vi "Create Process.vi"(8 "error in (no error)":errorcluster, 11 "Process Generator in":refnum<class "Process Generator.lvclass">) -> (0 "error out":errorcluster, 3 "Process Generator out":refnum<class "Process Generator.lvclass">)   [LabVIEW 2020, in "Process Generation.lvlib" / "Process Generator.lvclass"]
uses:
  Process Generator.lvclass
  Process Generator.lvclass/Process Generator.ctl
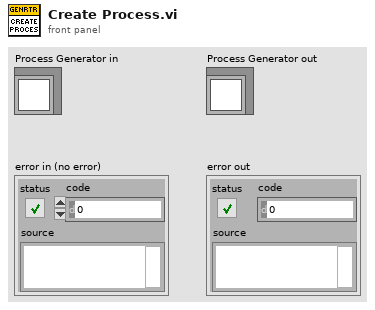
[diagram p1: front panel]
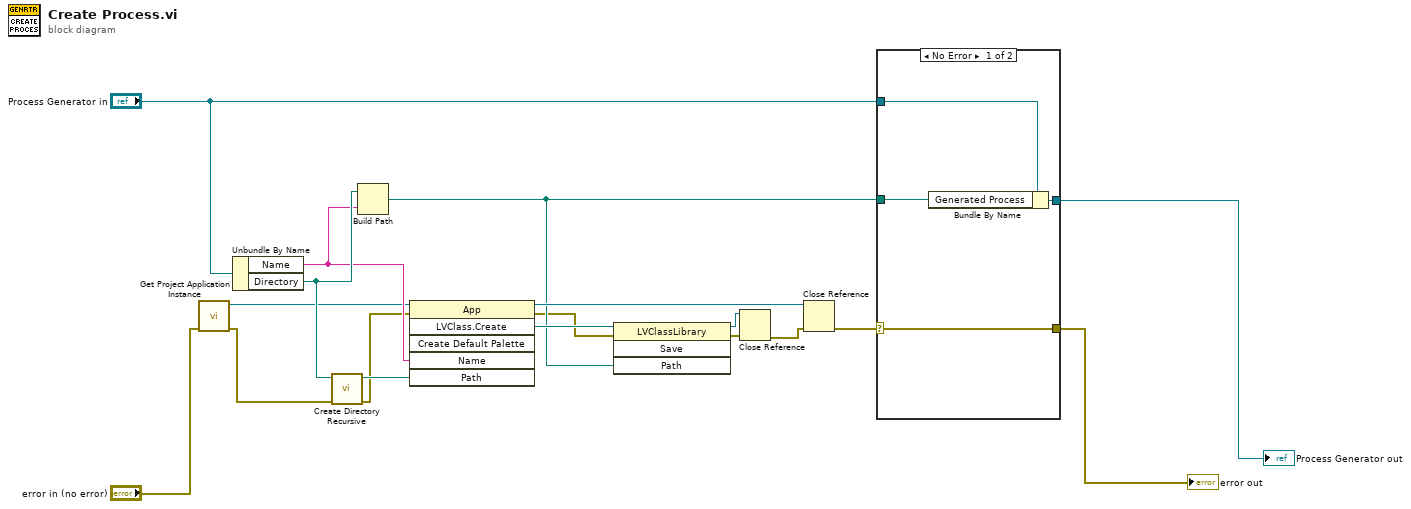
[diagram p0: block diagram]
diagram:
  n1 = call "Get Project Application Instance.vi"("error in (no error)"="error in (no error)") -> ("error out"=w10:errorcluster, "Application out"=w8:refnum<vi>)  [unwired: 9 in]
  n2 = Unbundle By Name("Process Generator in") -> ("Name"=w12:string, "Directory"=w13:path)
  n3 = call <vilib>:"Create Directory Recursive.vi"("error in (no error)"=w10, "directory"=w13) -> ("error out"=w7:errorcluster, "directory copy"=w18:path)  [unwired: 3 in, 1 out]
  n4 = Build Path(base path=w13, name or relative path=w12) -> (appended path=w5:path)
  n5 = invoke class="App" method="LVClass.Create"(reference=w8, error in=w7, "Name"=w12, "Path"=w18) -> (reference out=w15:refnum<vi>, error out=w2:errorcluster, "LVClass.Create"=w6:refnum<vi>)  [unwired: 2 in, 3 out]
  n6 = invoke class="LVClassLibrary" method="Save"(reference=w6, error in=w2, "Path"=w5) -> (reference out=w3:refnum<vi>, error out=w4:errorcluster)  [unwired: 1 in, 2 out]
  n7 = Close Reference(reference=w3, error in (no error)=w4) -> (error out=w1:errorcluster)
  n8 = Close Reference(reference=w15, error in (no error)=w1) -> (error out=w14:errorcluster)
  n9 = case shown="No Error" w14 {
    selector: w14 -> [w19 w23]
    tunnel: w5 -> [w22 _]
    tunnel: "Process Generator in" -> [w21 w24]
    tunnel: [w20 w24] -> w16
    tunnel: [w19 w23] -> w17
    frame No Error {
      n10 = Bundle By Name(cluster=w21, "Generated Process"=w22) -> (w20:refnum<class "Process Generator.lvclass">)
    }
    frame Error {
    }
  }
  "error out" <- w17
  "Process Generator out" <- w16
